vi "Set Endianness.vi"(7 "Message Flattener in":refnum<class "Message Flattener.lvclass">, 11 "bytes to read":i32) -> (3 "bytes to read":i32)   [LabVIEW 2020, in "Message Flattener.lvclass"]
doc: "Override this VI to change the endianness of the four-byte size value that is prepended to the serialized message. By default this value is big-endian."
uses:
  Message Flattener.lvclass
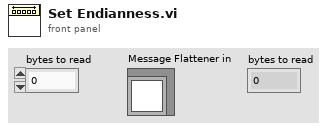
[diagram p1: front panel]
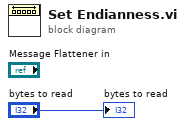
[diagram p0: block diagram]
diagram:
  "bytes to read" <- "bytes to read"
